vi "test ASK.vi"() -> ()   [LabVIEW 2019]
uses:
  <vilib>/addons/Modulation/Analog/support/mod_Set Error Source.vi
  <vilib>/addons/Modulation/Digital/General/MT Generate ASK system parameters (M).vi
  <vilib>/addons/Modulation/Digital/Support/Common/Validators/mod_Generate Filter Coefficients Validate.vi
  <vilib>/addons/Modulation/Digital/General/subVIs/mod_Generate Filter Coefficients.vi
  <vilib>/addons/Modulation/Analog/MT Upconvert Baseband (Real).vi
  <vilib>/addons/Modulation/Analog/MT Downconvert Passband (Real).vi
  <vilib>/express/express analysis/Spectral/Block/exnSpectralBlock spectral measurements RMS poly.vi
  <vilib>/express/express analysis/Spectral/Block/exnSpectralBlock spectral measurements RMS WFM.vi
  <vilib>/express/express analysis/Spectral/XNode/ExpressSpectralMeasurementsBlockNode.xnode
  <vilib>/addons/Modulation/niDMT.lvlib
  <vilib>/addons/Modulation/niAMT.lvlib
panel:
  in  "CRC":u8[](array[numeric])=[240, 210]
  out "measurements":T1 {"phase offset (deg)" format="%.2f"; "frequency drift (Hz)" format="%.2f"; "frequency offset (Hz)" format="%.2f"}
  out "Waveform Graph 5":cluster{"t0":dbl, "dt":dbl, "Y":dbl[]}(graph)
  out "Waveform Graph 4":cluster{"t0":dbl, "dt":dbl, "Y":dbl[]}(graph)
  out "output bit stream 2":i8[](array[numeric])
  out "Waveform Graph 3":cluster{"t0":dbl, "dt":dbl, "Y":dbl[]}(graph)
  out "output bit stream":i8[](array[numeric])
  out "Waveform Graph 2":waveform(dbl)(graph)
  out "Waveform Graph":cluster{"t0":dbl, "dt":dbl, "Y":dbl[]}(graph)
  in  "divider for bite rade":enum16{"32", "64", "128"}(ring)
  in  "bit rade":dbl
  in  "Carrier":dbl=13560.0
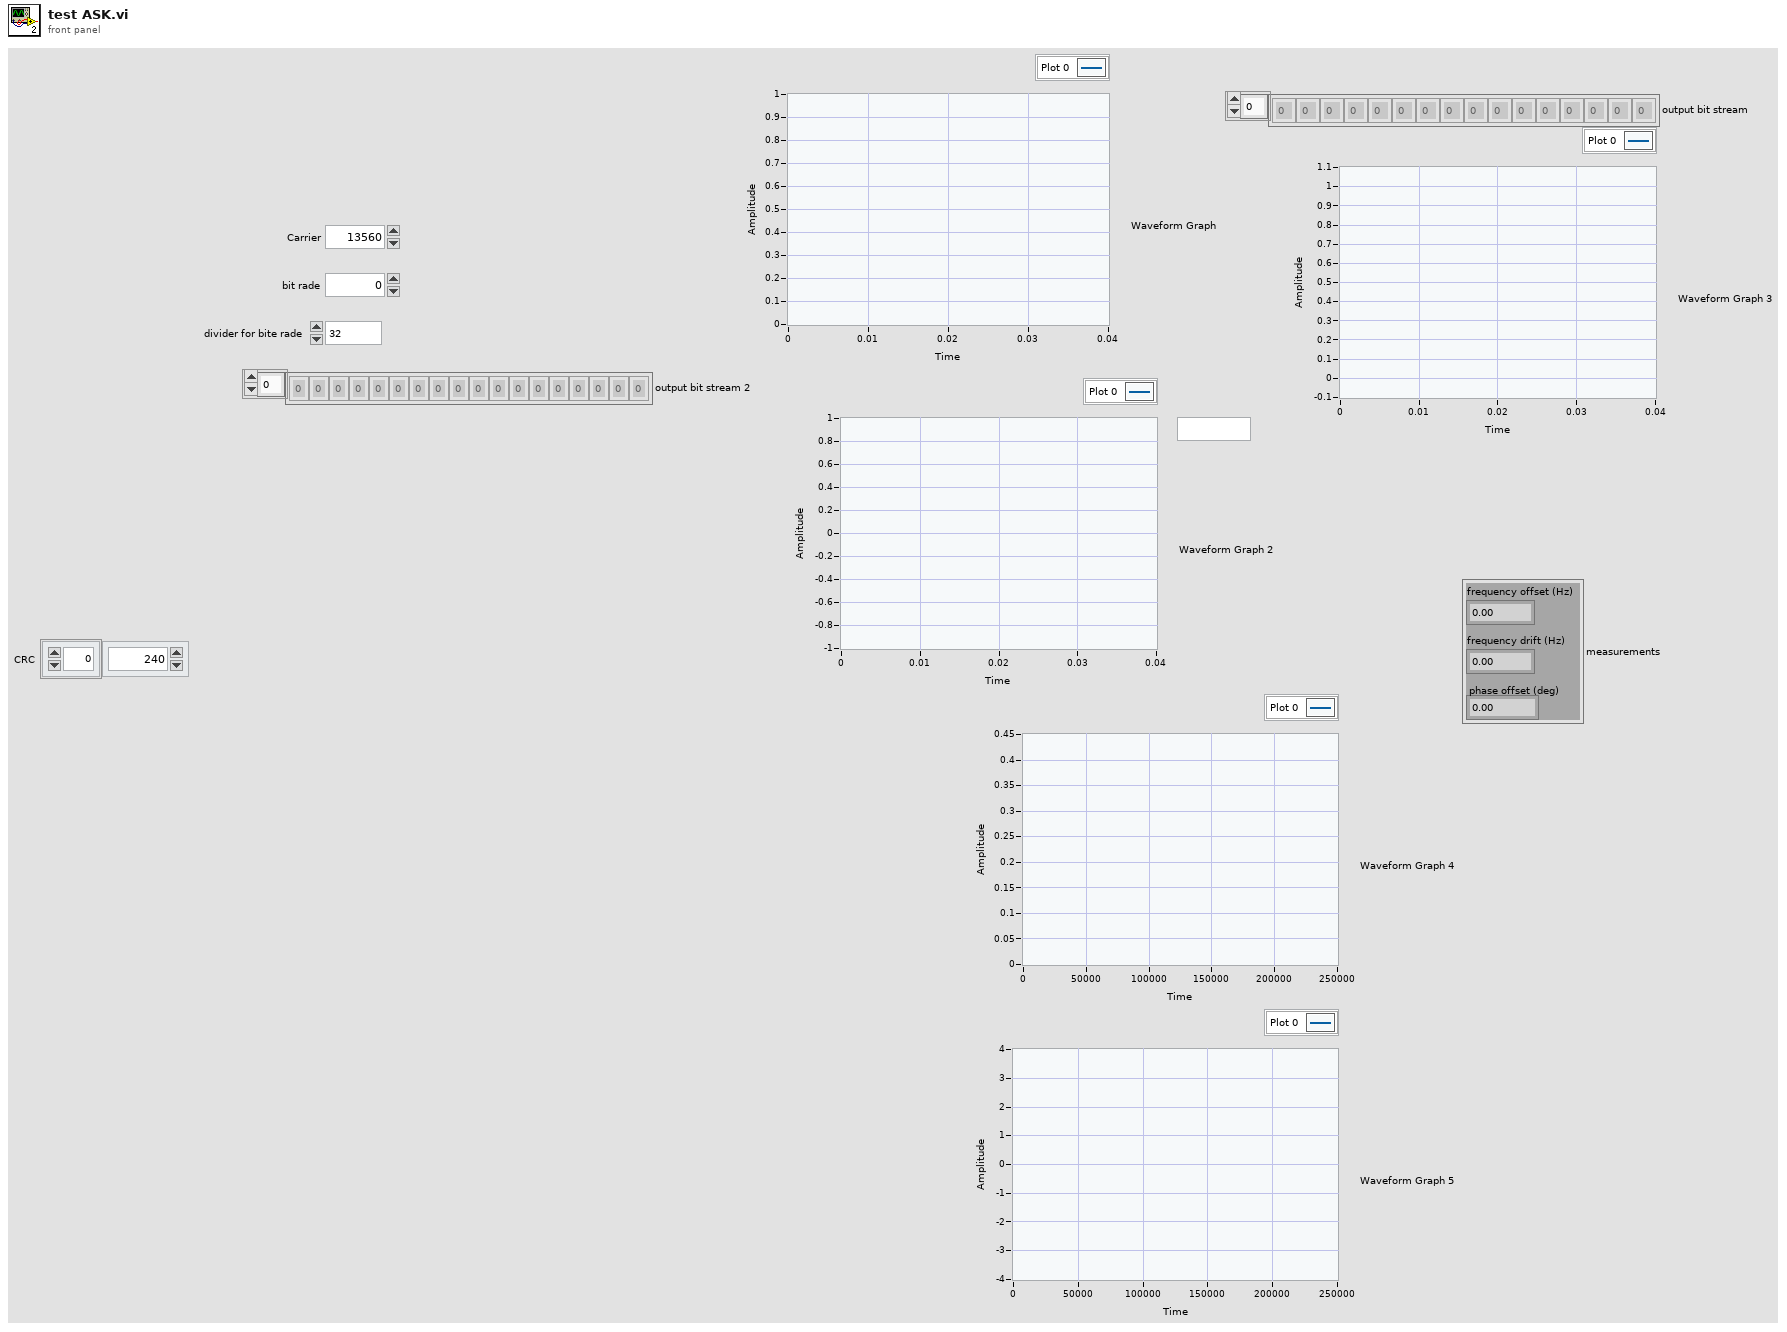
[diagram p1: front panel]
types:
  T1 = cluster{"frequency offset (Hz)":dbl, "frequency drift (Hz)":dbl, "phase offset (deg)":dbl}
  T2 = enum16{"none", "Raised Cosine", "Root Raised Cos", "Gaussian"}
  T3 = enum16{"FSK", "PSK", "QAM", "MSK", "PAM", "ASK", "CPM"}
  T4 = cluster{"averaging mode":u16, "weighting mode":u16, "number of averages":u32}
  T5 = cluster{"dB On (F)":bool, "unwrap phase (F)":bool, "convert to degree (F)":bool}
  T6 = cluster{"samples per symbol (16)":i32, "symbol map":cdb[]}
  T7 = typedef "niAMT.lvlib/Complex Data Waveform.ctl" = cluster{"t0":dbl, "dt":dbl, "Y":cdb[]}
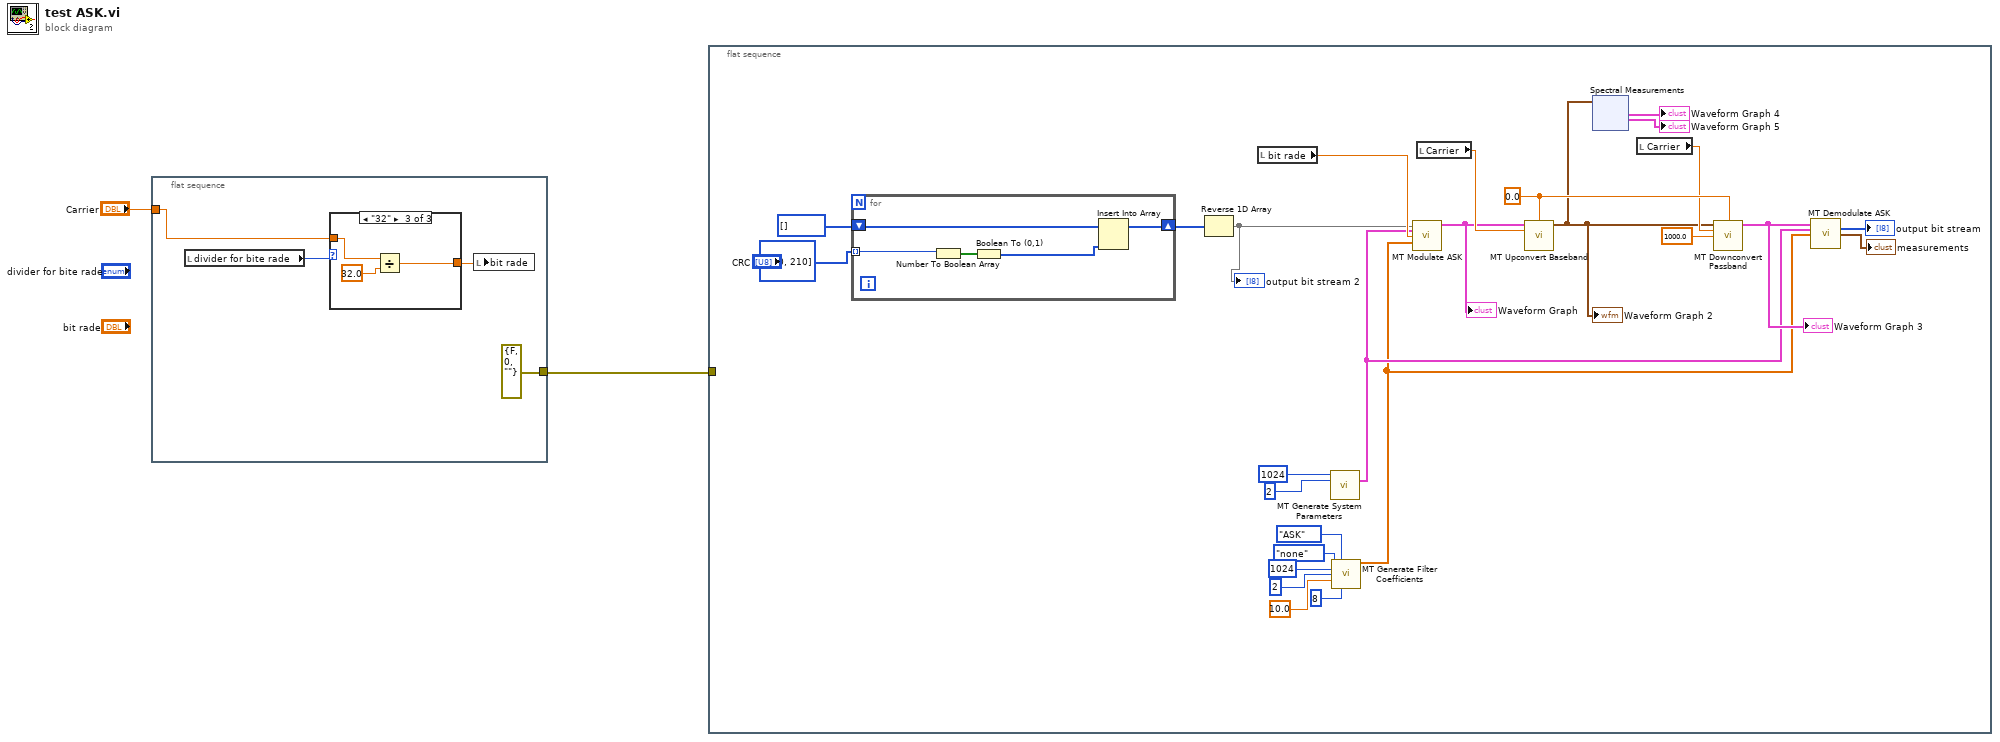
[diagram p0: block diagram]
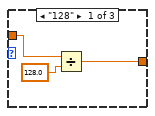
[diagram p2: hidden frame]
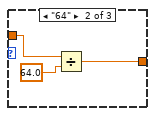
[diagram p3: hidden frame]
diagram:
  n1 = flat-sequence {
    tunnel: "Carrier" -> [w5]
    tunnel: [errorcluster {"status"=FALSE, "code"=0, "source"=""} ("error in (no error)")] -> w1
    frame #0 {
      n2 = local read "divider for bite rade"() -> (w6:enum16{"32", "64", "128"})
      n3 = case shown="\"32\"" w6 {
        tunnel: w5 -> [w9 w12 w15]
        tunnel: [w7 w10 w13] -> w4
        frame "128" {
          n4 = Divide(x=w9, y=128.0) -> (x/y=w7:dbl)
        }
        frame "64" {
          n5 = Divide(x=w12, y=64.0) -> (x/y=w10:dbl)
        }
        frame "32" {
          n6 = Divide(x=w15, y=32.0) -> (x/y=w13:dbl)
        }
      }
      n7 = local write "bit rade"(w4) -> ()
    }
  }
  n8 = flat-sequence {
    tunnel: w1 -> [_]
    frame #0 {
      w28 = 0.0 ("initial phase (deg)")
      n9 = for {
        tunnel: u8[] [240, 210] ("CRC") -> [w56] mode=indexing
        shift-right: [w53] -> w41
        shift-left: i16[] [] -> [w52]
        n10 = Number To Boolean Array(number=w56) -> (Boolean array=w55:bool[])
        n11 = Boolean To (0,1)(Boolean=w55) -> (0, 1=w54:i16[])
        n12 = Insert Into Array(array=w52, new element=w54) -> (w53:i16[])  [unwired: 1 in]
      }
      n13 = Reverse 1D Array(array=w41) -> (reversed array=w17:i16[])
      "output bit stream 2" <- w17
      n14 = local read "bit rade"() -> (w34:dbl)
      n15 = call-poly <vilib>:"MT Generate System Parameters.vi"("samples per symbol (16)"=1024, "M-ASK (2)"=2) -> ("ASK system parameters"=w24:T6)  [unwired: 11 in, 2 out]
      n16 = call <vilib>:"MT Generate Filter Coefficients.vi"("pulse shaping filter (none)"=T2."none", "modulation type"=T3."ASK", "pulse shaping samples per symbol (16)"=1024, "matched samples per symbol (16)"=2, "filter parameter"=10.0, "filter length (symbols)"=8) -> ("pulse shaping filter coefficients"=w23:dbl[])  [unwired: 7 in, 2 out]
      n17 = call <vilib>:"MT Modulate ASK.vi"("input bit stream"=w17, "ASK system parameters"=w24, "symbol rate (Hz)"=w34, "pulse shaping filter coefficients"=w23) -> ("output complex waveform"=w29:T7)  [unwired: 9 in, 2 out]
      "Waveform Graph" <- w29
      n18 = local read "Carrier"() -> (w30:dbl)
      n19 = call-poly <vilib>:"MT Upconvert Baseband.vi"("baseband waveform (complex)"=w29, "initial phase (deg)"=w28, "carrier frequency (Hz)"=w30) -> ("passband waveform"=w20:waveform(dbl))  [unwired: 11 in, 1 out]
      "Waveform Graph 2" <- w20
      n20 = xnode "Spectral Measurements"("Signals"=w20) -> ("FFT - (RMS)"=→"Waveform Graph 4":cluster{"f0":dbl, "df":dbl, "magnitude":dbl[]}, "Phase"=→"Waveform Graph 5":cluster{"f0":dbl, "df":dbl, "phase":dbl[]})  [unwired: 1 in, 1 out]
      n21 = local read "Carrier"() -> (w27:dbl)
      n22 = call-poly <vilib>:"MT Downconvert Passband.vi"("Waveform"=w20, "initial phase (deg)"=w28, "carrier frequency (Hz)"=w27, "passband bandwidth (Hz)"=1000.0) -> ("downconverted waveform (complex baseband)"=w25:T7)  [unwired: 8 in, 3 out]
      "Waveform Graph 3" <- w25
      n23 = call <vilib>:"MT Demodulate ASK.vi"("input complex waveform"=w25, "ASK system parameters"=w24, "matched filter coefficients"=w23) -> ("output bit stream"=→"output bit stream":i8[], "measurements"=→"measurements":T1)  [unwired: 8 in, 3 out]
    }
  }
